vi "Build_task.vi"(7 "index":i32, 8 "error in":errorcluster, 11 "Builder in":refnum<class "Builder.lvclass">) -> (0 "error out":errorcluster, 2 "Generated files":path[](array[path]), 3 "Builder out":refnum<class "Builder.lvclass">)   [LabVIEW 2021, in "App-Builder Library.lvlib" / "Builder.lvclass"]
uses:
  Builder.lvclass
  Builder.lvclass/Builder.ctl
  <vilib>/AppBuilder/AB_API_Simple/Build (path).vi
  <vilib>/AppBuilder/AB_API_Simple/NI_App_Builder_API.lvlib
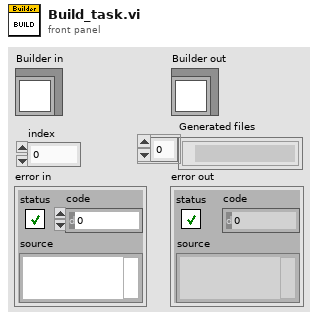
[diagram p1: front panel]
types:
  T1 = typedef "App-Builder Library.lvlib/Builder.lvclass/Build specification.ctl" = cluster{"target name":string, "Build specification":string, "Project Path":path, "Build Object type":T2}
  T2 = typedef "App-Builder Library.lvlib/Builder.lvclass/Build object type.ctl" = enum16{"EXE", "RT EXE", "Deployable Packed"}
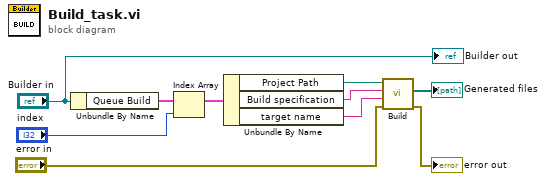
[diagram p0: block diagram]
diagram:
  n1 = Unbundle By Name("Builder in") -> ("Queue Build"=w10:T1[])
  n2 = Index Array(array=w10, index="index") -> (element=w4:T1)
  n3 = Unbundle By Name(w4) -> ("Project Path"=w7:path, "Build specification"=w6:string, "target name"=w5:string)
  n4 = call-poly <vilib>:"Build.vi"("error in (no error)"="error in", "Name of target (My Computer)"=w5, "Name of build specification (if empty: build all)"=w6, "Path to project"=w7) -> ("error out"=→"error out":errorcluster, "Generated files"=→"Generated files":path[])  [unwired: 6 in]
  "Builder out" <- "Builder in"
